vi "draw.vi"(8 "error in (no error)":errorcluster, 11 "Gerade in":refnum<class "Gerade.lvclass">) -> (0 "error out":errorcluster, 2 "Line":cluster{"x":dbl[], "y":dbl[]}, 3 "Gerade out":refnum<class "Gerade.lvclass">)   [LabVIEW 2019, in "Gerade.lvclass"]
uses:
  Gerade.lvclass
  Gerade.lvclass/Gerade.ctl
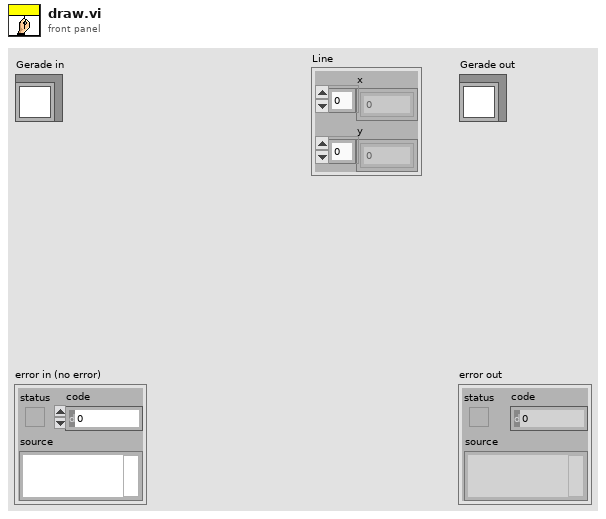
[diagram p1: front panel]
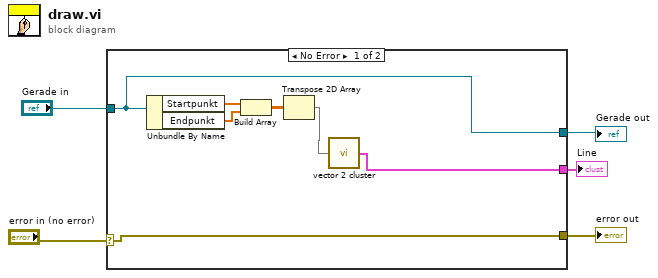
[diagram p0: block diagram]
diagram:
  n1 = case shown="No Error" "error in (no error)" {
    selector: "error in (no error)" -> [w12 w14]
    tunnel: [w12 w14] -> w4
    tunnel: "Gerade in" -> [w9 w13]
    tunnel: [w9 w13] -> w2
    tunnel: [w7 _] -> w1
    frame No Error {
      n2 = Unbundle By Name(w9) -> ("Startpunkt"=w11:dbl[], "Endpunkt"=w10:dbl[])
      n3 = Build Array(w11, w10) -> (w8:dbl[][])
      n4 = Transpose 2D Array(2D array=w8) -> (transposed array=w6:dbl[][])
      n5 = call "vector 2 cluster.vi"("coordinates"=w6) -> (0:w7:cluster{"x":dbl[], "y":dbl[]})
    }
    frame Error {
    }
  }
  "error out" <- w4
  "Gerade out" <- w2
  "Line" <- w1
